vi "call library.vi"() -> ()   [LabVIEW 2023]
uses:
  modules/cmh-library/Message Queue/Enqueue Message.vi
  <extravilib>/ChannelInstances/Messenger-t'Message Queue.lvlib-Message Cluster.ctl'/Write.vi
  <extravilib>/ChannelInstances/Messenger-t'Message Queue.lvlib-Message Cluster.ctl'/Write With Abort.vi
  <extravilib>/ChannelInstances/Messenger-t'Message Queue.lvlib-Message Cluster.ctl'/Instantiate.vi
  <extravilib>/ChannelInstances/Messenger-t'Message Queue.lvlib-Message Cluster.ctl'/Endpoint.vi
  Nanotec Controller.lvlib
  modules/cmh-library/Message Queue.lvlib
panel:
  out "error out":errorcluster
  in  "error in":errorcluster
  # "THIS VI EXISTS ONLY BECAUSE CHANNELS ON THE CONNECTOR NEED TO BE CONNECTED.\nUSE THIS VI IN ORDER TO USE THE NANOTEC CONTROLLER IN STANDALONE"
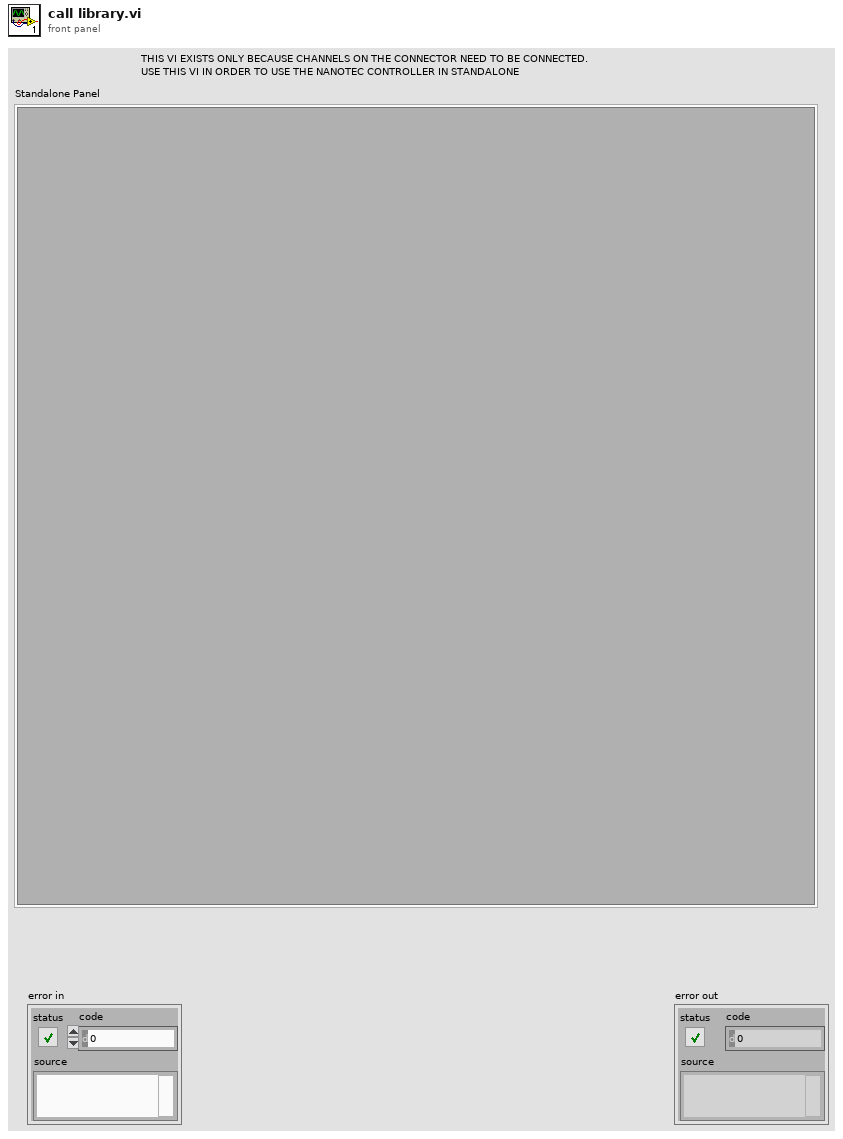
[diagram p1: front panel]
types:
  T1 = typedef "Messenger-t'Message Queue.lvlib-Message Cluster.ctl'.lvlib/))Channel.ctl" = refnum<queue>
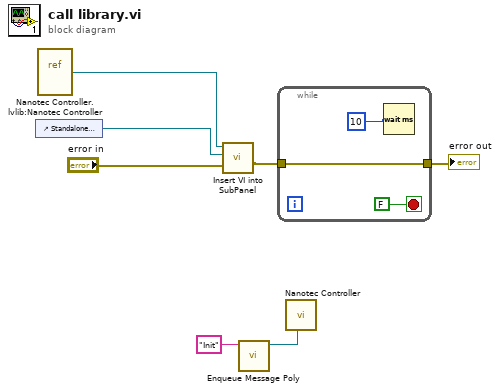
[diagram p0: block diagram]
diagram:
  n1 = control-ref of="Standalone Panel"() -> (w6:refnum<vi>)
  n2 = vi-ref "Nanotec Controller.lvlib:Nanotec Controller.vi"() -> (w7:refnum<vi>)
  n3 = call <userlib>:"Insert VI into SubPanel.vi"("error in"="error in", "SubPnl Ref"=w6, "VI in"=w7) -> ("error out"=w4:errorcluster)  [unwired: 8 in]
  n4 = call-poly "Enqueue Message Poly.vi"("Message"="Init") -> ("channel"=w2:T1)  [unwired: 10 in]
  n5 = while {
    tunnel: [w10] -> w3
    tunnel: w4 -> [w10]
    stop <- FALSE stop-if-true
    n6 = Wait (ms)(milliseconds to wait=u32 10) -> ()  [unwired: 1 out]
  }
  "error out" <- w3
  n7 = call "Nanotec Controller.vi"("remote"=w2) -> ()  [unwired: 11 in]
